vi "MCL Iss Configure Polarity.vi"(9 "handle":i32, 10 "mode":i32, 11 "clock":i32) -> (3 "function return":i32)   [LabVIEW 2017, in "Madlib.lvlib"]
doc: "MADLIB_API int MCL_IssConfigurePolarity(int clock, int mode, int handle);"
uses:
  Madlib.lvlib
  Madlib.dll
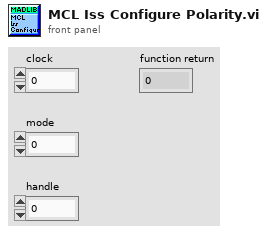
[diagram p1: front panel]
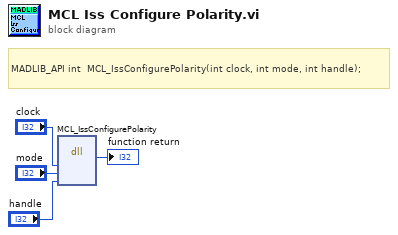
[diagram p0: block diagram]
diagram:
  # "MADLIB_API\tint\t\tMCL_IssConfigurePolarity(int clock, int mode, int handle);"
  n1 = dll-call lib="C:/Users/francesco/dev/pump-probe/Piezo/lvlib/Madlib.*" fn="MCL_IssConfigurePolarity"("clock"="clock", "mode"="mode", "handle"="handle") -> (→"function return":i32)  [unwired: 6 in, 2 out]
